vi "build_popup.vi"() -> (2 "y_vals":dbl[](array[numeric])=[0.0, 1.0, 2.0, 3.0, 4.0, 5.0, 6.0, 7.0, 8.0, 9.0, 10.0], 3 "cancelled":bool)   [LabVIEW 2017, in "tools.lvlib"]
uses:
  tools.lvlib
  core/build_pars.ctl
panel:
  out "init":bool
  in  "build_pars":T1={"build using"=enum."start: step: num", "start"=0.0, "step"=1.0, "end"=10.0, "num"=11, "rescale"=1.0} {"rescale" format="%#_6p"; "end" format="%#.8g"; "start" format="%#_8g"; "step" format="%#_8g"}
  in  "Cancel":bool
  in  "OK Button":bool
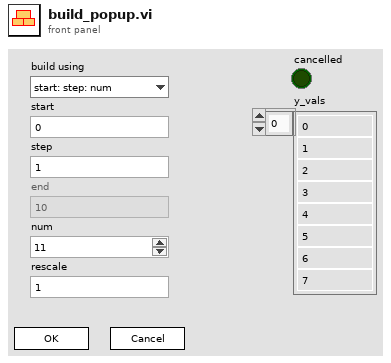
[diagram p1: front panel]
types:
  T1 = typedef "tools.lvlib/build_pars.ctl" = cluster{"build using":enum16{"start: end: num", "start: step: end", "start: step: num"}, "start":dbl, "step":dbl, "end":dbl, "num":i32, "rescale":dbl}
  T2 = enum8{"Enabled", "Disabled", "Disabled and Grayed Out"}
  T3 = enum16{"start: end: num", "start: step: end", "start: step: num"}
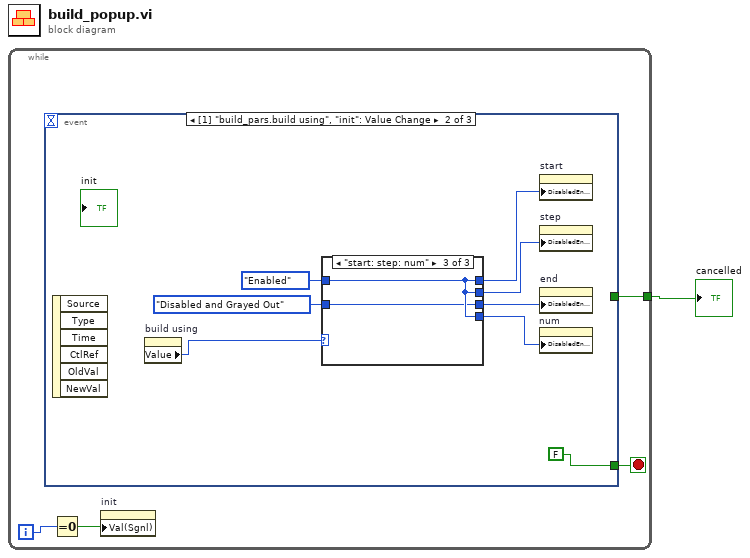
[diagram p0: block diagram]
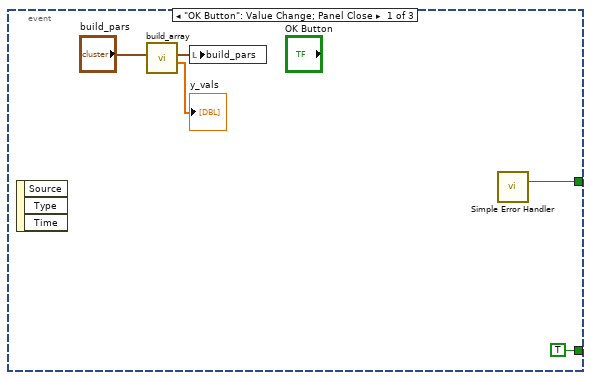
[diagram p2: hidden frame]
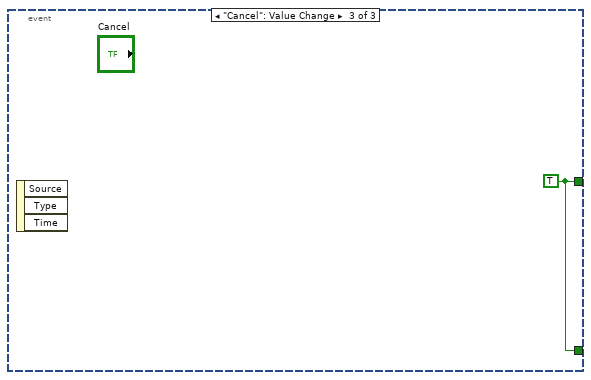
[diagram p5: hidden frame]
diagram:
  n1 = while {
    tunnel: [w5] -> w1
    i -> [w3]
    stop <- w4 stop-if-true
    n2 = event shown="[1] \"build_pars.build using\", \"init\": Value Change" {
      selector: _ -> [_ _ _]
      dyn-events: _ -> [_ _ _]
      timeout: _ -> [_ _ _]
      tunnel: [w10 _ w25] -> w5
      tunnel: [TRUE ("Cancel") FALSE w25] -> w4
      event "OK Button": Value Change; Panel Close {
        n3 = event-data() -> ()  [unwired: 1 in, 3 out]
        n4 = call "build_array.vi"("settings IN"="build_pars") -> ("values"=→"y_vals":dbl[], "settings OUT"=w7:T1)  [unwired: 9 in]
        n5 = local write "build_pars"(w7) -> ()
        n6 = call <vilib>:"Simple Error Handler.vi"() -> ("error?"=w10:bool)  [unwired: 5 in, 4 out]
      }
      event "init": Value Change {
        n7 = event-data() -> ()  [unwired: 1 in, 6 out]
        n8 = property on="build using" class="Enum (strict)"() -> ("Value"=w11:T3)  [unwired: 2 in, 2 out]
        n9 = case shown="\"start: step: num\"" w11 {
          tunnel: T2."Enabled" ("Disabled") -> [w20 w22 w24]
          tunnel: [w20 w22 w23] -> w14
          tunnel: [w20 w22 w24] -> w16
          tunnel: [w19 w22 w24] -> w15
          tunnel: [w20 w21 w24] -> w13
          tunnel: T2."Disabled and Grayed Out" ("Disabled") -> [w19 w21 w23]
          frame "start: end: num", Default {
          }
          frame "start: step: end" {
          }
          frame "start: step: num" {
          }
        }
        n10 = property on="start" class="DigNum (strict)"("DisabledEnum"=w16) -> ()  [unwired: 2 in, 2 out]
        n11 = property on="step" class="DigNum (strict)"("DisabledEnum"=w15) -> ()  [unwired: 2 in, 2 out]
        n12 = property on="end" class="DigNum (strict)"("DisabledEnum"=w14) -> ()  [unwired: 2 in, 2 out]
        n13 = property on="num" class="DigNum (strict)"("DisabledEnum"=w13) -> ()  [unwired: 2 in, 2 out]
      }
      event "Cancel": Value Change {
        w25 = TRUE ("Cancel")
        n14 = event-data() -> ()  [unwired: 1 in, 3 out]
      }
    }
    n15 = Equal To 0?(x=w3) -> (x = 0?=w2:bool)
    n16 = property on="init" class="Bool (strict)"("Val(Sgnl)"=w2) -> ()  [unwired: 2 in, 2 out]
  }
  "cancelled" <- w1
